vi "ServiceChannels.Status.Set.vi"(4 "Buffer?":bool, 5 "Status Lookup":variant, 6 "Type":T1, 7 "Service Channels Status Ref":T2, 8 "error in (no error)":errorcluster, 9 "Status":bool, 11 "ID":u32) -> (0 "error out":errorcluster)   [LabVIEW 2019, in "Diagnostics Addon Engine.lvlib"]
uses:
  Diagnostics Addon Engine.lvlib
  <vilib>/NI/NIVS Inline Async API/_Data Access Engine/Data Access Engine/Types/Write.DVR.ctl
  <vilib>/NI/NIVS Inline Async API/_Data Access Engine/Access Type Classes/Write/Write.lvclass
  Shared/Types/Type.ctl
  Shared/Types/ServiceChannels.LookupType.ctl
  <vilib>/NI/NIVS Inline Async API/_Data Access Engine/Access Type Classes/Write/Write.lvclass/Write.ctl
  <vilib>/NI/NIVS Inline Async API/_Data Access Engine/Data Access Engine/Methods/Write.Data.Buffer.vi
  <vilib>/NI/NIVS Inline Async API/_Data Access Engine/Data Access Engine/Methods/Write.Data.vi
  <vilib>/NI/NIVS Inline Async API/_Data Access Engine/Access Type Classes/Write/Write.Buffer.vi
  <vilib>/NI/NIVS Inline Async API/_Data Access Engine/Access Type Classes/Write/Write.ProcessData.vi
  <vilib>/NI/NIVS Inline Async API/_Data Access Engine/Access Type Classes/Write/Write.Commit.vi
  <vilib>/NI/NIVS Inline Async API/_Data Access Engine/Data Access Engine/Data Access Engine.lvclass
  Shared/Diagnostics Addon Shared.lvlib
  <vilib>/Utility/SystemLogging/NI_SystemLogging.lvlib
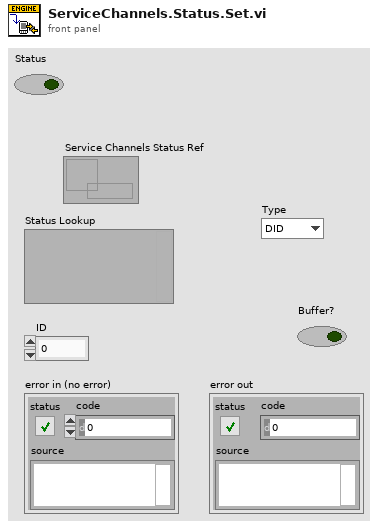
[diagram p1: front panel]
types:
  T1 = typedef "Diagnostics Addon Shared.lvlib/Type.ctl" = enum16{"DID", "CDID", "PID", "CPID", "Read Memory", "Write Memory", "IO Control", "Routine Start", "Routine Request", "Routine Stop", "User Defined", "DTC Control", "Clear DTCs", "Read DTCs", "Start DTCs", "DTC Change Count", "Tester Present", "Unlock ECU", "Reset ECU", "Diag Session Control", "Communication Control", "DPID Control", "Poll Control", "Diag CAN Control"}
  T2 = typedef "Data Access Engine.lvlib/Data Access Engine.lvclass/Write.DVR.ctl" = refnum<data-value>
  T3 = enum16{"Output/Write", "Input/Read", "Input/ReadWrite"}
  T4 = typedef "Diagnostics Addon Shared.lvlib/ServiceChannels.LookupType.ctl" = cluster{"Offset":i32}
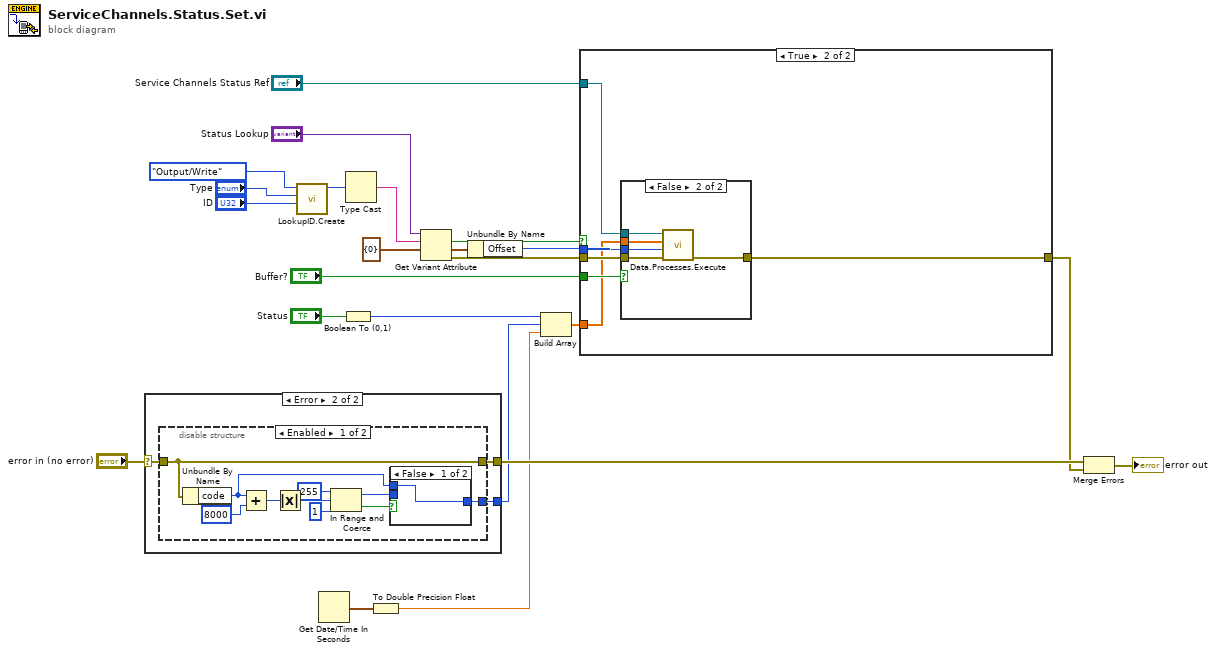
[diagram p0: block diagram]
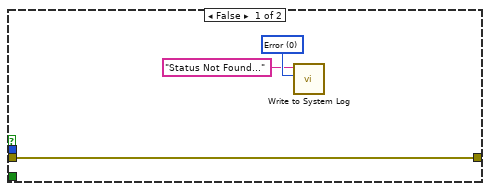
[diagram p2: hidden frame]
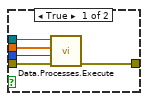
[diagram p3: hidden frame]
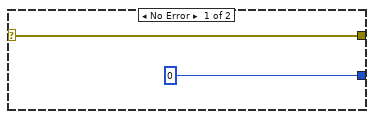
[diagram p4: hidden frame]
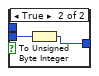
[diagram p5: hidden frame]
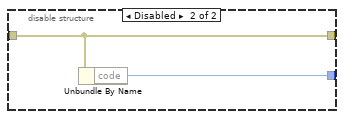
[diagram p6: hidden frame]
diagram:
  n1 = case shown="Error" "error in (no error)" {
    selector: "error in (no error)" -> [w24 w27]
    tunnel: [0 w28] -> w10
    tunnel: [w24 w26] -> w13
    frame No Error {
    }
    frame Error {
      n2 = disable-structure shown="Enabled" {
        disable-tunnel: [w32 w43] -> w28
        disable-tunnel: w27 -> [w29 w42]
        disable-tunnel: [w29 w42] -> w26
        frame Enabled {
          n3 = Unbundle By Name(w29) -> ("code"=w30:i32)
          n4 = Add(x=w30, y=8000) -> (x+y=w37:i32)
          n5 = Absolute Value(x=w37) -> (abs(x)=w36:i32)
          n6 = In Range and Coerce(upper limit=255, x=w36, lower limit=1) -> (coerced(x)=w31:i32, In Range?=w33:bool)
          n7 = case shown="False" w33 {
            tunnel: [w39 w40] -> w32
            tunnel: w31 -> [_ w41]
            tunnel: w30 -> [w39 _]
            frame False {
            }
            frame True {
              n8 = To Unsigned Byte Integer(number=w41) -> (unsigned 8bit integer=w40:u8)
            }
          }
        }
        frame Disabled {
          n9 = Unbundle By Name(w42) -> ("code"=w43:i32)
        }
      }
    }
  }
  n10 = call "LookupID.Create.vi"("Serivce ID"="ID", "Service Type"="Type", "Direction"=T3."Output/Write") -> ("Result"=w5:u64)  [unwired: 8 in]
  n11 = Get Date/Time In Seconds() -> (seconds since 1Jan1904=w9:timestamp)
  n12 = Boolean To (0,1)(Boolean="Status") -> (0, 1=w1:i16)
  n13 = Type Cast(x=w5) -> (*(type *) &x=w18:string)  [unwired: 1 in]
  n14 = To Double Precision Float(number=w9) -> (double precision float=w8:dbl)
  n15 = Get Variant Attribute(Variant="Status Lookup", name=w18, default value (empty Variant)=T4 {"Offset"=0} ("cluster")) -> (found=w16:bool, value=w20:T4, error out=w15:errorcluster)  [unwired: 1 in, 1 out]
  n16 = Unbundle By Name(w20) -> ("Offset"=w17:i32)
  n17 = Build Array(w1, w10, w8) -> (w7:dbl[])
  n18 = case shown="True" w16 {
    tunnel: "Service Channels Status Ref" -> [_ w51]
    tunnel: [w46 w50] -> w12
    tunnel: w17 -> [_ w52]
    tunnel: "Buffer?" -> [_ w49]
    tunnel: w15 -> [w46 w48]
    tunnel: w7 -> [_ w47]
    frame False {
      w45 = 0 items=["Error", "Warning", "Informational"] ("severity")
      n19 = call <vilib>:"Write to System Log.vi"("severity"=w45, "message"="Status Not Found..." ("Message")) -> ()  [unwired: 9 in, 1 out]
    }
    frame True {
      n20 = case shown="False" w49 {
        tunnel: w52 -> [w57 w62]
        tunnel: w47 -> [w56 w61]
        tunnel: w51 -> [w55 w58]
        tunnel: w48 -> [w54 w60]
        tunnel: [w53 w59] -> w50
        frame True {
          n21 = call-poly <vilib>:"Data.Processes.Execute.vi"("error in (no error)"=w54, "Offset"=w57, "Values"=w56, "Ref"=w55) -> ("error out"=w53:errorcluster)  [unwired: 7 in]
        }
        frame False {
          n22 = call-poly <vilib>:"Data.Processes.Execute.vi"("error in (no error)"=w60, "Offset"=w62, "Values"=w61, "Ref"=w58) -> ("error out"=w59:errorcluster)  [unwired: 7 in]
        }
      }
    }
  }
  n23 = Merge Errors(w13, w12) -> (→"error out":errorcluster)
